vi "画垂线.vi"(9 "Caliper Results (点到直线距离)":sgl[][](array[numeric]), 10 "点":cluster{"X":sgl, "Y":sgl}[](array[cluster]), 11 "引用句柄输入":T1) -> (3 "点到线距离":sgl[][](array[numeric]))   [LabVIEW 2014]
uses:
  <vilib>/vision/Image Controls.llb/IMAQ Image.ctl
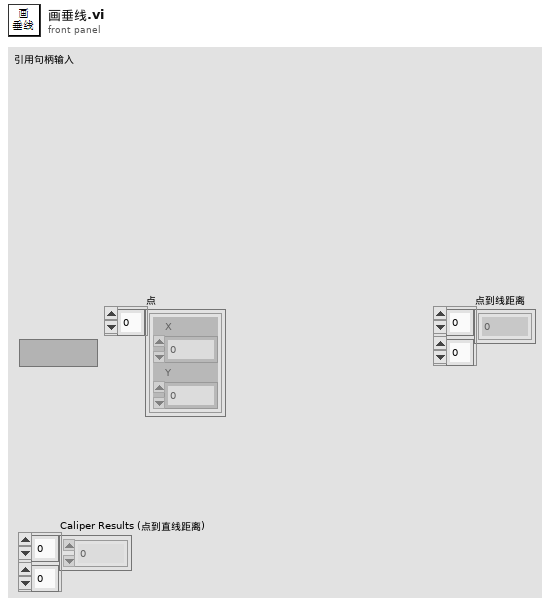
[diagram p1: front panel]
types:
  T1 = typedef "IMAQ Image.ctl" = refnum<image>
  T2 = cluster{"output string":sgl, "output string":sgl}
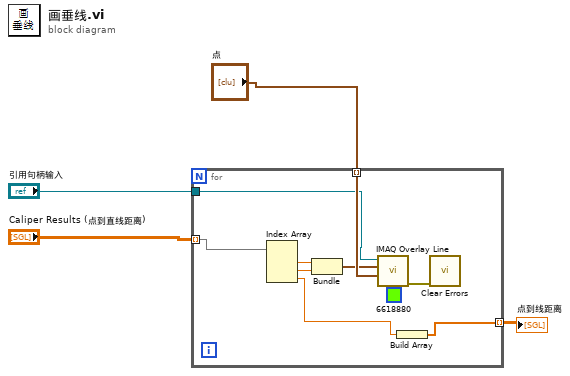
[diagram p0: block diagram]
diagram:
  n1 = for {
    tunnel: "点" -> [w14] mode=indexing
    tunnel: "引用句柄输入" -> [w13]
    tunnel: "Caliper Results (点到直线距离)" -> [w7] mode=indexing
    tunnel: [w5] -> w2 mode=indexing
    n2 = Index Array(array=w7) -> (element #1=w8:sgl, element #2=w9:sgl, element #3=w6:sgl)  [unwired: 3 in]
    n3 = Bundle("output string"=w8, "output string"=w9) -> (w12:T2)  [unwired: 1 in]
    n4 = call "IMAQ Overlay Line"("Color"=u32 6618880, "End Point"=w14, "Start Point"=w12, "Image"=w13) -> ("error out"=w11:errorcluster)  [unwired: 6 in, 1 out]
    n5 = Build Array(w6) -> (w5:sgl[])
    n6 = call <vilib>:"Clear Errors.vi"("error in (no error)"=w11) -> ()  [unwired: 5 in, 2 out]
  }
  "点到线距离" <- w2
